vi "bufferToArrays.vi"(8 "error in (no error)":errorcluster, 10 "BufferString":string, 11 "ElectrometerController in":refnum<class "ElectrometerController.lvclass">) -> (0 "error out":errorcluster, 1 "time":dbl[](array[numeric]), 2 "value":dbl[](array[numeric]), 3 "ElectrometerController out":refnum<class "ElectrometerController.lvclass">, 4 "count":dbl[](array[numeric]))   [LabVIEW 2016, in "ElectrometerController.lvclass"]
uses:
  ElectrometerController.lvclass
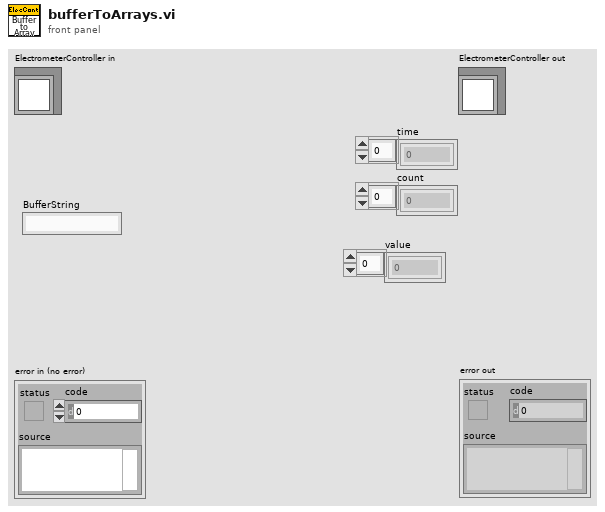
[diagram p1: front panel]
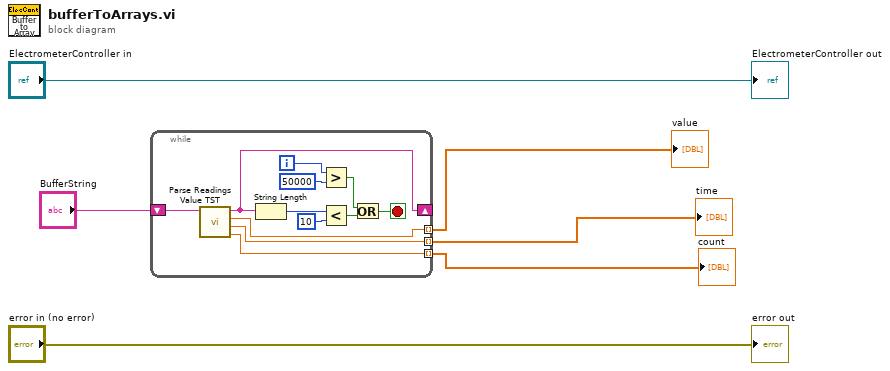
[diagram p0: block diagram]
diagram:
  n1 = while {
    shift-right: [w15] -> _
    shift-left: "BufferString" -> [w18]
    tunnel: [w17] -> w4 mode=indexing
    tunnel: [w16] -> w3 mode=indexing
    tunnel: [w7] -> w2 mode=indexing
    i -> [w10]
    stop <- w8 stop-if-true
    n2 = call "Parse Readings Value TST.vi"("Readings"=w18) -> ("count"=w7:dbl, "Time"=w16:dbl, "Measurement"=w17:dbl, "Remain Readings"=w15:string)  [unwired: 7 in]
    n3 = String Length(string=w15) -> (length=w14:i32)
    n4 = Greater?(x=w10, y=50000) -> (0:w11:bool)
    n5 = Less?(x=w14, y=10) -> (x < y?=w12:bool)
    n6 = Or(x=w11, y=w12) -> (x .or. y?=w8:bool)
  }
  "value" <- w4
  "time" <- w3
  "count" <- w2
  "error out" <- "error in (no error)"
  "ElectrometerController out" <- "ElectrometerController in"
